vi "Create Reference Locals.vi"(5 "Sequence Context":refnum<k7>) -> (0 "error out":errorcluster)   [LabVIEW 2013, in "MiscHelperVIs.lvlib"]
uses:
  MiscHelperVIs.lvlib
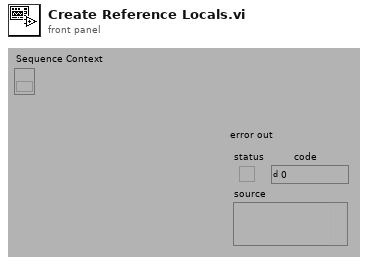
[diagram p1: front panel]
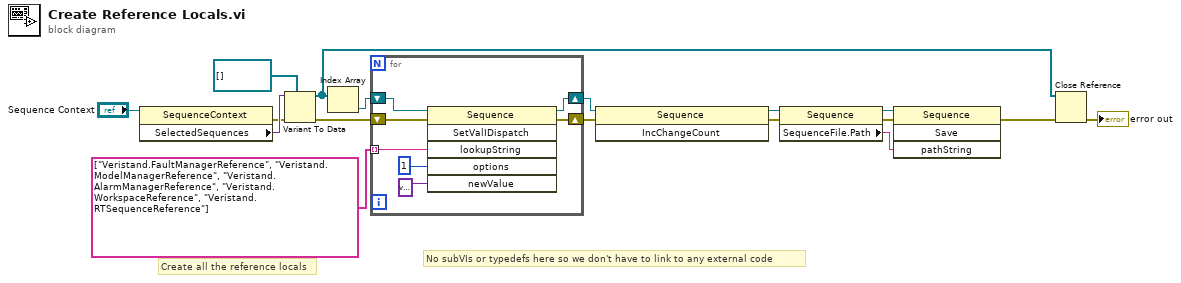
[diagram p0: block diagram]
diagram:
  # "No subVIs or typedefs here so we don't have to link to any external code"
  # "Create all the reference locals"
  n1 = property class="SequenceContext"(reference="Sequence Context") -> (error out=w12:errorcluster, "SelectedSequences"=w16:variant)  [unwired: 1 in, 1 out]
  n2 = Variant To Data(error in=w12, type=refnum<k7>[] [], Variant=w16) -> (data=w9:refnum<k7>[], error out=w11:errorcluster)
  n3 = Index Array(array=w9) -> (element=w7:refnum<k7>)  [unwired: 1 in]
  n4 = for {
    shift-right: [w23] -> w13
    shift-left: w11 -> [w24]
    tunnel: string[] ["Veristand.FaultManagerReference", "Veristand.ModelManagerReference", "Veristand.AlarmManagerReference", "Veristand.WorkspaceReference", "Veristand.RTSequenceReference"] -> [w22] mode=indexing
    shift-right: [w19] -> w10
    shift-left: w7 -> [w18]
    n5 = invoke class="Sequence" method="SetValIDispatch"(reference=w18, error in=w24, "lookupString"=w22, "options"=1, "newValue"=variant) -> (reference out=w19:refnum<k7>, error out=w23:errorcluster)  [unwired: 1 in, 4 out]
  }
  n6 = invoke class="Sequence" method="IncChangeCount"(reference=w10, error in=w13) -> (reference out=w6:refnum<k7>, error out=w5:errorcluster)  [unwired: 1 in, 1 out]
  n7 = property class="Sequence"(reference=w6, error in=w5) -> (reference out=w3:refnum<k7>, error out=w4:errorcluster, "SequenceFile.Path"=w2:string)
  n8 = invoke class="Sequence" method="Save"(reference=w3, error in=w4, "pathString"=w2) -> (error out=w1:errorcluster)  [unwired: 1 in, 3 out]
  n9 = Close Reference(reference=w9, error in (no error)=w1) -> (error out=→"error out":errorcluster)
